vi "Any file exists.vi"(8 "Error In":errorcluster, 11 "Files":path[](array[path])) -> (0 "Error Out":errorcluster, 3 "Any file exists?":bool)   [LabVIEW 2015]
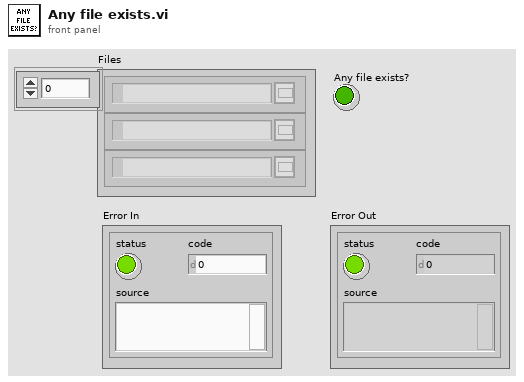
[diagram p1: front panel]
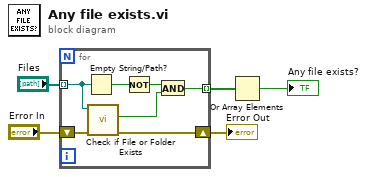
[diagram p0: block diagram]
diagram:
  n1 = for {
    tunnel: "Files" -> [w12] mode=indexing
    shift-right: [w7] -> w3
    shift-left: "Error In" -> [w8]
    tunnel: [w6] -> w2 mode=indexing
    n2 = Empty String/Path?(string/path=w12) -> (empty?=w11:bool)
    n3 = call <vilib>:"Check if File or Folder Exists.vi"("error in (no error)"=w8, "path"=w12) -> ("error out"=w7:errorcluster, "file or folder exists?"=w9:bool)  [unwired: 7 in, 1 out]
    n4 = Not(x=w11) -> (.not. x?=w10:bool)
    n5 = And(x=w10, y=w9) -> (x .and. y?=w6:bool)
  }
  "Error Out" <- w3
  n6 = Or Array Elements(Boolean array=w2) -> (logical OR=→"Any file exists?":bool)
